vi "Module Top Level.vi"   [LabVIEW 2018, in "RT - Analysis.lvlib"]
doc: "This is the top level VI for this module. It uses a queue for communications and is stopped user a user event. The general architecture is similar to a simple queued message handler.\n\nThe VIs associated with this module are organized in a LabVIEW Library."
uses:
  RT - Analysis.lvlib
panel:
  # "RT - Analysis"
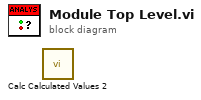
[diagram p0: block diagram]
diagram:
  n1 = call "Calc Calculated Values 2.vi"() -> ()  [unwired: 10 in, 2 out]
